vi "Test_ParseCommandFromAnswer.vi"() -> ()   [LabVIEW 2023]
uses:
  <vilib>/addons/_JKI Toolkits/Caraya/classes/Assert/Assert Equal Value and Type_Variant.vi
  <vilib>/addons/_JKI Toolkits/Caraya/classes/Assert/Assert Not Error.vi
  <vilib>/addons/_JKI Toolkits/Caraya/classes/Test/Test.lvclass
  <vilib>/addons/_JKI Toolkits/Caraya/classes/Assert/Assert.lvclass
  Classes/Communicator/Communicator.lvclass
panel:
  out "JSON values":string
  out "JSON keys":string="ccd_getChipSize"
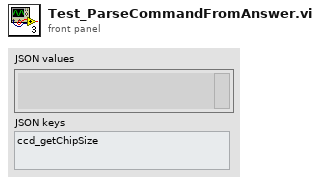
[diagram p1: front panel]
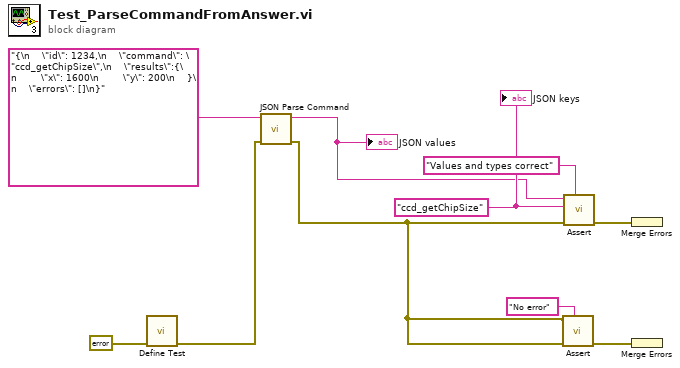
[diagram p0: block diagram]
diagram:
  w7 = "ccd_getChipSize" ("JSON keys")
  n1 = call <vilib>:"Define Test.vi"("error in (no error)"=errorcluster {"status"=FALSE, "code"=0, "source"=""}) -> ("error out"=w3:errorcluster)  [unwired: 9 in, 1 out]
  n2 = call "JSON Parse Command.vi"("error in (no error)"=w3, "JSON command"="{\n    \"id\": 1234,\n    \"command\": \"ccd_getChipSize\",\n    \"results\":{\n        \"x\": 1600\n        \"y\": 200\n    }\n    \"errors\": []\n}") -> ("error out"=w2:errorcluster, "returned command"=w1:string)  [unwired: 7 in, 1 out]
  "JSON values" <- w1
  n3 = call-poly <vilib>:"Assert.vi"("Label"="No error" ("Label (VI Title)"), "error in (no error)"=w2, "Not Error?"=w2) -> ("error out"=w5:errorcluster)  [unwired: 7 in, 1 out]
  n4 = call-poly <vilib>:"Assert.vi"("Label"="Values and types correct" ("Label (VI Title)"), "error in (no error)"=w2, "Y"=w7, "X"=w1) -> ("error out"=w8:errorcluster)  [unwired: 6 in, 1 out]
  n5 = Merge Errors(w8) -> ()  [unwired: 1 out]
  n6 = Merge Errors(w5) -> ()  [unwired: 1 out]
  "JSON keys" <- w7
